vi "Show Data Logger.vi"(8 "error in":errorcluster, 11 "Study Actor in":refnum<class "Study Actor.lvclass">) -> (0 "error out":errorcluster, 3 "Study Actor out":refnum<class "Study Actor.lvclass">)   [LabVIEW 2023, in "Study Actor.lvlib" / "Study Actor.lvclass"]
uses:
  Study Actor.lvclass
  Study Actor.lvclass/Study Actor.ctl
  Series/ISeries Actor/ISeries Actor Messages/Show Data Logger Msg/Show Data Logger Msg.lvclass
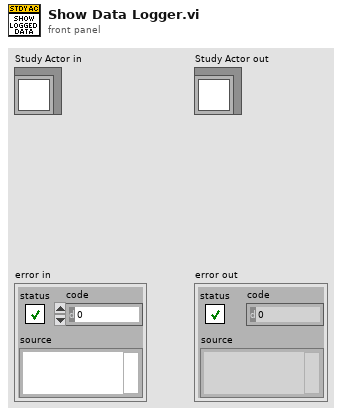
[diagram p1: front panel]
types:
  T1 = map{string, refnum<class "Message Enqueuer.lvclass">}
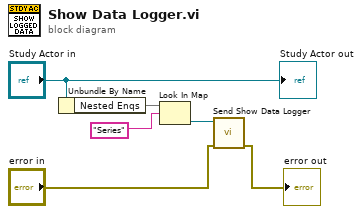
[diagram p0: block diagram]
diagram:
  n1 = Unbundle By Name("Study Actor in") -> ("Nested Enqs"=w5:T1)
  n2 = Look In Map(map=w5, key="Series") -> (value=w3:refnum<class "Message Enqueuer.lvclass">)  [unwired: 1 in, 1 out]
  n3 = call "Send Show Data Logger.vi"("error in (no error)"="error in", "Message Enqueuer"=w3) -> ("error out"=→"error out":errorcluster)  [unwired: 8 in, 1 out]
  "Study Actor out" <- "Study Actor in"
